vi "Temperature FGV.vi"(8 "error in (no error)":errorcluster, 10 "Temp. Input":dbl, 11 "Tag Name":string) -> (0 "error out":errorcluster, 2 "History Data":T1(array[cluster]))   [LabVIEW 2023]
uses:
  8fdf3798-820e-43b9-bbcf-a8150b0dfc24.vi
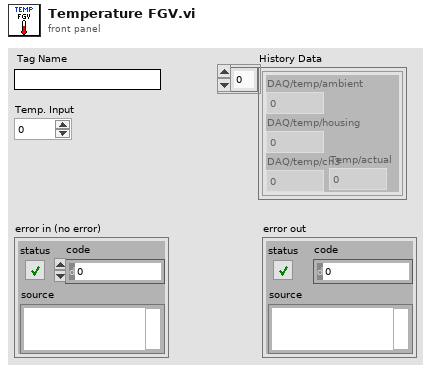
[diagram p1: front panel]
types:
  T1 = cluster{"DAQ/temp/ambient":dbl, "DAQ/temp/housing":dbl, "DAQ/temp/ch3":dbl, "Temp/actual":dbl}[]
  T2 = cluster{"DAQ/temp/ambient":dbl, "DAQ/temp/housing":dbl, "DAQ/temp/ch3":dbl, "Temp/actual":dbl}
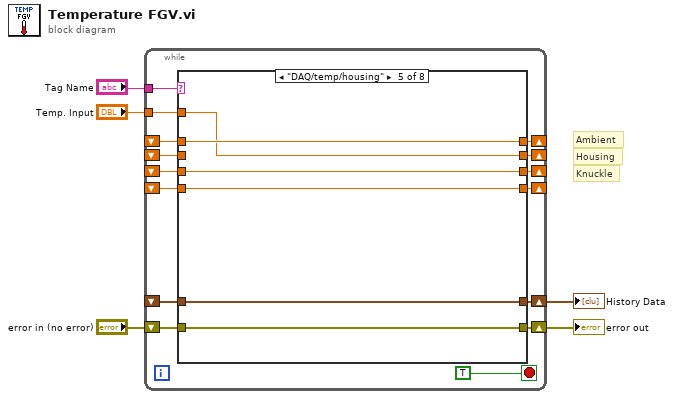
[diagram p0: block diagram]
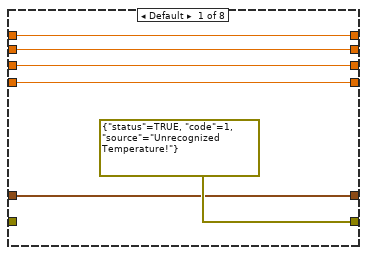
[diagram p2: hidden frame]
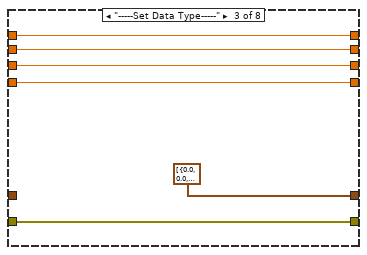
[diagram p4: hidden frame]
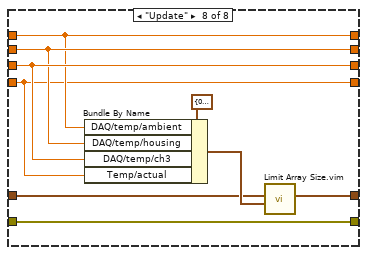
[diagram p8: hidden frame]
diagram:
  # "Knuckle"
  # "Housing"
  # "Ambient"
  n1 = while {
    tunnel: "Tag Name" -> [w16]
    shift-right: [w14] -> w2
    shift-left: _ -> [w15]
    shift-right: [w18] -> w4
    shift-left: "error in (no error)" -> [w19]
    shift-right: [w13] -> _
    shift-left: _ -> [w17]
    shift-right: [w12] -> _
    shift-left: _ -> [w9]
    shift-right: [w11] -> _
    shift-left: _ -> [w10]
    tunnel: "Temp. Input" -> [w8]
    shift-right: [w6] -> _
    shift-left: _ -> [w7]
    stop <- TRUE stop-if-true
    n2 = case shown="\"DAQ/temp/housing\"" w16 {
      tunnel: w19 -> [_ w32 w38 w44 w50 w56 w62 w71]
      tunnel: [errorcluster {"status"=TRUE, "code"=1, "source"="Unrecognized Temperature!"} ("error constant") w32 w38 w44 w50 w56 w62 w71] -> w18
      tunnel: w17 -> [w24 w30 w36 _ w48 w55 w61 w67]
      tunnel: w15 -> [w25 w31 _ w41 w47 w54 w59 w64]
      tunnel: [w25 w31 T1 [{"DAQ/temp/ambient"=0.0, "DAQ/temp/housing"=0.0, "DAQ/temp/ch3"=0.0, "Temp/actual"=0.0}] ("History Data") w41 w47 w54 w59 w63] -> w14
      tunnel: [w24 w30 w36 w40 w48 w55 w61 w67] -> w13
      tunnel: [w22 w28 w34 w42 w49 w52 w57 w69] -> w12
      tunnel: [w23 w29 w35 w43 w46 w51 w60 w68] -> w11
      tunnel: w10 -> [w23 w29 w35 w43 _ w51 w60 w68]
      tunnel: w9 -> [w22 w28 w34 w42 w49 _ w57 w69]
      tunnel: w8 -> [_ _ _ w40 w46 w52 w58 _]
      tunnel: w7 -> [w21 w27 w33 w39 w45 w53 _ w66]
      tunnel: [w21 w27 w33 w39 w45 w53 w58 w66] -> w6
      frame Default {
      }
      frame "" {
      }
      frame "-----Set Data Type-----" {
      }
      frame "DAQ/temp/ambient" {
      }
      frame "DAQ/temp/housing" {
      }
      frame "DAQ/temp/ch3" {
      }
      frame "Temp/actual" {
      }
      frame "Update" {
        n3 = Bundle By Name(cluster=T2 {"DAQ/temp/ambient"=0.0, "DAQ/temp/housing"=0.0, "DAQ/temp/ch3"=0.0, "Temp/actual"=0.0}, "DAQ/temp/ambient"=w67, "DAQ/temp/housing"=w68, "DAQ/temp/ch3"=w69, "Temp/actual"=w66) -> (w65:T2)
        n4 = call "Limit Array Size.vim"("Numeric"=w65, "Array in"=w64) -> ("Array out"=w63:T1)  [unwired: 5 in]
      }
    }
  }
  "error out" <- w4
  "History Data" <- w2
